vi "createScriptEvent.vi"(8 "error in (no error)":errorcluster, 11 "ScriptEditorV2 in":refnum<class "ScriptEditorV2.lvclass">) -> (0 "error out":errorcluster, 3 "ScriptEditorV2 out":refnum<class "ScriptEditorV2.lvclass">)   [LabVIEW 2009, in "Views.lvlib" / "ScriptEditor.lvlib" / "ScriptEditorV2.lvclass"]
uses:
  ScriptEditorV2.lvclass
  EventEditor/ActionEditor/ActionEditor.lvclass
  ScriptEditorV2.lvclass/ScriptEditorV2.ctl
  Tools/Scripting/ScriptingEvent/ScriptEventList/ScriptEventList.lvclass
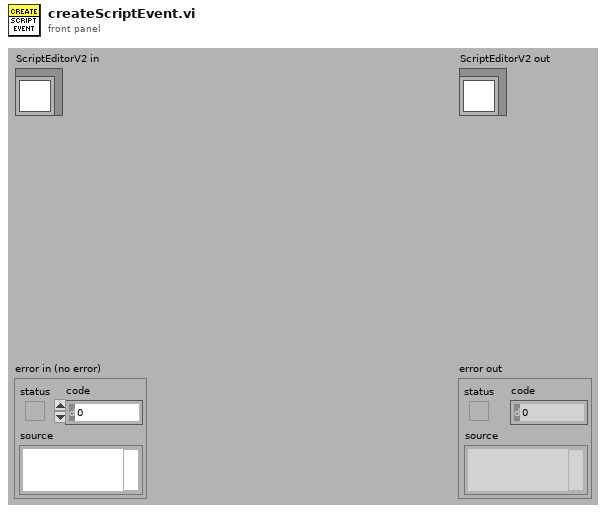
[diagram p1: front panel]
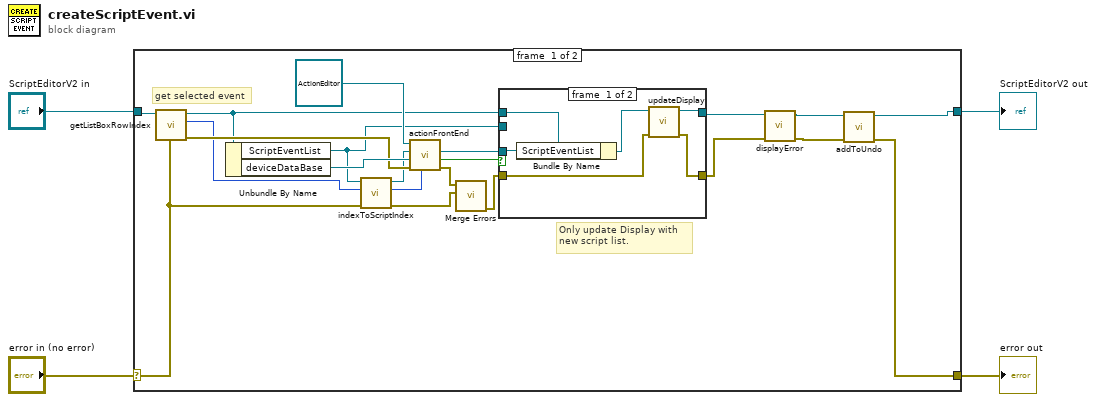
[diagram p0: block diagram]
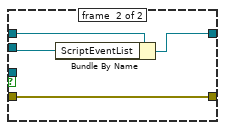
[diagram p2: hidden frame]
diagram:
  n1 = case shown="No Error" "error in (no error)" {
    selector: "error in (no error)" -> [w12 w37]
    tunnel: [w5 w37] -> w3
    tunnel: [w7 w36] -> w1
    tunnel: "ScriptEditorV2 in" -> [w25 w36]
    frame #0 {
      # "get selected event"
      # "Only update Display with\nnew script list."
      n2 = call "getListBoxRowIndex.vi"("error in (no error)"=w12, "ScriptEditorV2 in"=w25) -> ("error out"=w23:errorcluster, "rowIndex"=w16:i32, "ScriptEditorV2 out"=w21:refnum<class "ScriptEditorV2.lvclass">)  [unwired: 7 in]
      n3 = Unbundle By Name(w21) -> ("ScriptEventList"=w14:refnum<class "ScriptEventList.lvclass">, "deviceDataBase"=w24:refnum<class "deviceDataBase.lvclass">)
      n4 = call "indexToScriptIndex.vi"("error in (no error)"=w12, "sequencedIndex"=w16, "ScriptEventList in"=w14) -> ("error out"=w9:errorcluster, "indexScriptEvent"=w15:i32, "ScriptEventList out"=w13:refnum<class "ScriptEventList.lvclass">)  [unwired: 6 in]
      n5 = call-dynamic "actionFrontEnd.vi"("index"=w15, "error in (no error)"=w23, "deviceDataBase"=w24, "ScriptEventList"=w13, "ActionEditor in"=refnum<class "ActionEditor.lvclass"> refnum ("Views.lvlib:SciptEditor.lvlib:ActionEditor.lvclass")) -> ("error out"=w11:errorcluster, "canceled"=w20:bool, "ScriptEventList out"=w19:refnum<class "ScriptEventList.lvclass">)  [unwired: 3 in, 1 out]
      n6 = call <vilib>:"Merge Errors.vi"("error in 2 (no error)"=w9, "error in 1 (no error)"=w11) -> ("error out"=w10:errorcluster)  [unwired: 5 in]
      n7 = case shown="False" w20 {
        tunnel: w21 -> [w30 w34]
        tunnel: [w28 w33] -> w18
        tunnel: w10 -> [w27 w32]
        tunnel: w19 -> [w31 _]
        tunnel: w14 -> [_ w35]
        tunnel: [w26 w32] -> w17
        frame #0 {
          n8 = Bundle By Name(cluster=w30, "ScriptEventList"=w31) -> (w29:refnum<class "ScriptEditorV2.lvclass">)
          n9 = call "updateDisplay.vi"("error in (no error)"=w27, "ScriptEditorV2 in"=w29) -> ("error out"=w26:errorcluster, "ScriptEditorV2 out"=w28:refnum<class "ScriptEditorV2.lvclass">)  [unwired: 8 in]
        }
        frame #1 {
          n10 = Bundle By Name(cluster=w34, "ScriptEventList"=w35) -> (w33:refnum<class "ScriptEditorV2.lvclass">)
        }
      }
      n11 = call "displayError.vi"("error in (no error)"=w17, "ScriptEditorV2 in"=w18) -> ("error out"=w6:errorcluster, "ScriptEditorV2 out"=w8:refnum<class "ScriptEditorV2.lvclass">)  [unwired: 8 in]
      n12 = call "addToUndo.vi"("error in (no error)"=w6, "ScriptEditorV2 in"=w8) -> ("error out"=w5:errorcluster, "ScriptEditorV2 out"=w7:refnum<class "ScriptEditorV2.lvclass">)  [unwired: 8 in]
    }
    frame #1 {
    }
  }
  "error out" <- w3
  "ScriptEditorV2 out" <- w1
